vi "PIDinC 17.vi"(0 "Gain Schedule":cluster{dbl, dbl, dbl, dbl, dbl, dbl}, 1 "D":dbl, 2 "Time":dbl, 3 "Integral in":dbl, 4 "prev in":dbl, 6 "I":dbl, 7 "x in":dbl, 8 "P2":dbl, 9 "dt":dbl, 10 "P":dbl, 11 "I2":dbl, 12 "Set Point":dbl, 13 "PV":dbl, 14 "Total Time":dbl, 16 "D2":dbl) -> (15 "Integral out":dbl, 17 "MV":dbl, 18 "prev out":dbl, 19 "x out":dbl)   [LabVIEW 2011]
panel:
  out "Ti":dbl
  out "Kp":dbl
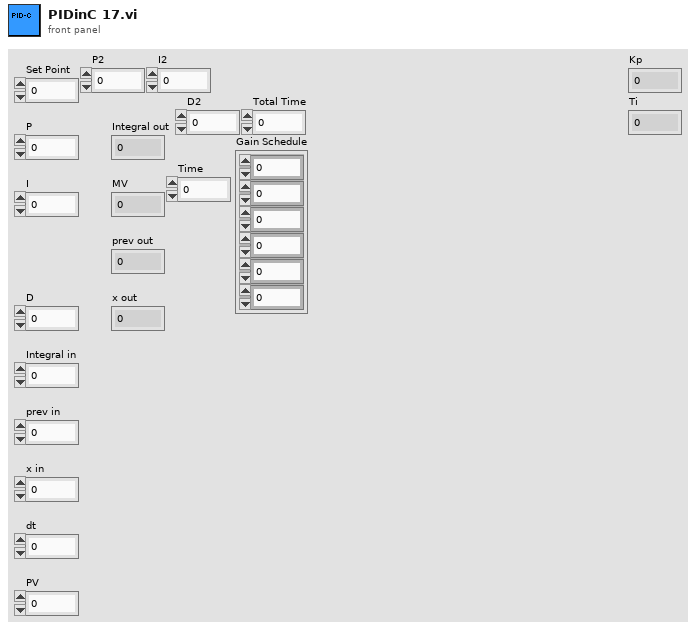
[diagram p1: front panel]
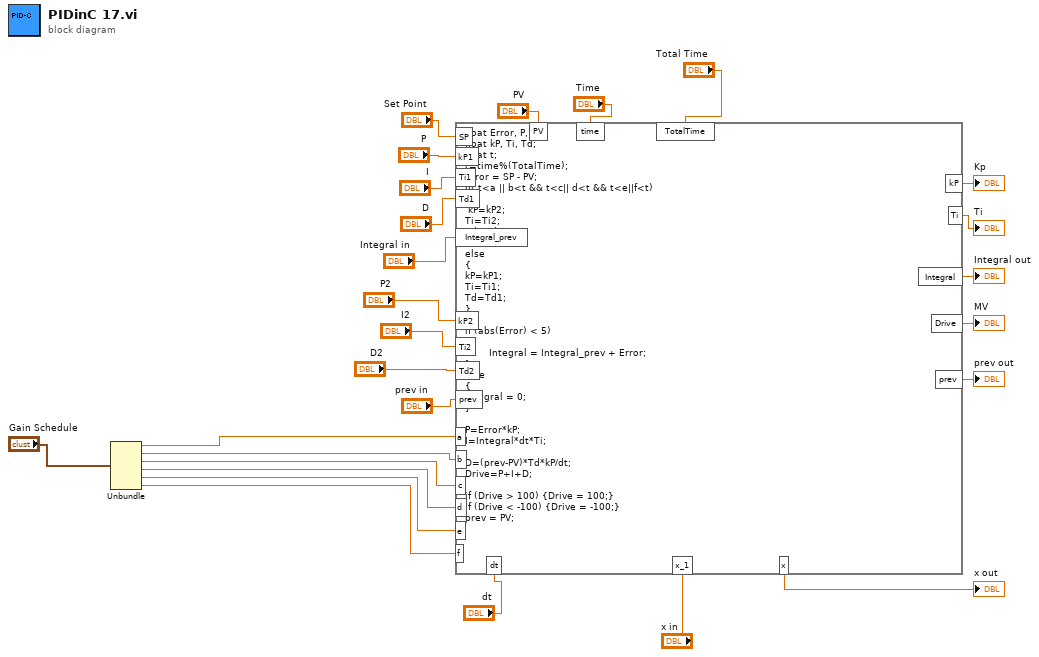
[diagram p0: block diagram]
diagram:
  n1 = Unbundle("Gain Schedule") -> (w5:dbl, w6:dbl, w4:dbl, w3:dbl, w2:dbl, w1:dbl)
  n2 = formula code="float Error, P, I,D;\nfloat kP, Ti, Td;\nfloat t;\nt=time%(TotalTime);\nError = SP - PV; \nif( t<a || b<t && t<c|| d<t && t<e||f<t)\n{\n kP=kP2;\nTi=Ti2;\nTd=Td2;\n}\nelse\n{\nkP=kP1;\nTi=Ti1;\nTd=Td1;\n}\n               \nif (abs(Error) < 5)\n{          \n        Integral = Integral_prev + Error;\n}      \nelse\n{\nIntegral = 0;\n}  \n\nP=Error*kP;\nI=Integral*dt*Ti;  \n\nD=(prev-PV)*Td*kP/dt;\nDrive=P+I+D;\n        \nif (Drive > 100) {Drive = 100;}      \nif (Drive < -100) {Drive = -100;} \nprev = PV;"("SP"="Set Point", "kP1"="P", "Ti1"="I", "Td1"="D", "PV"="PV", "dt"="dt", "x_1"="x in", "Integral_prev"="Integral in", "prev"="prev in", "TotalTime"="Total Time", "time"="Time", "kP2"="P2", "Ti2"="I2", "Td2"="D2", "a"=w5, "b"=w6, "c"=w4, "d"=w3, "e"=w2, "f"=w1) -> ("x"=→"x out":dbl, "Integral"=→"Integral out":dbl, "Drive"=→"MV":dbl, "prev"=→"prev out":dbl, "kP"=→"Kp":dbl, "Ti"=→"Ti":dbl)
